vi "OEE_SCREEN_2_update_graph_hourly_data.vi"(11 "SQL_raw_data_out":T1) -> ()   [LabVIEW 2019]
uses:
  FGV/SQL_raw_data/OEE_SQL_raw_data.ctl
  FGV/FGV_SCREEN_2_graph_hourly/FGV_SCREEN_2_graph_hourly.ctl
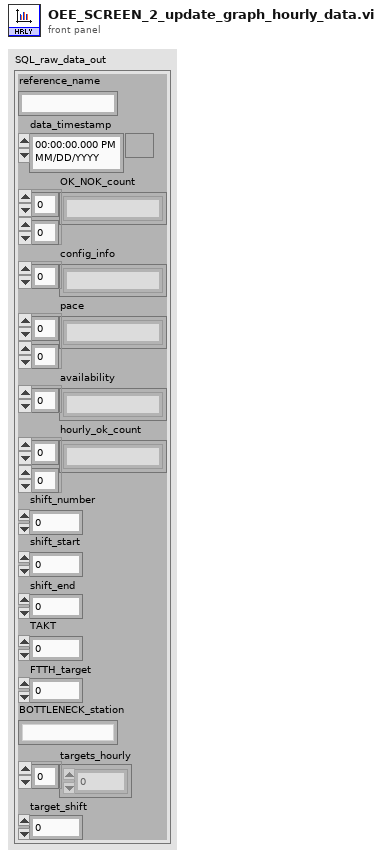
[diagram p1: front panel]
types:
  T1 = typedef "OEE_SQL_raw_data.ctl" = cluster{"reference_name":string, "data_timestamp":timestamp, "OK_NOK_count":string[][], "config_info":string[], "pace":string[][], "availability":string[], "hourly_ok_count":string[][], "shift_number":i8, "shift_start":i8, "shift_end":i8, "TAKT":u16, "FTTH_target":u16, "BOTTLENECK_station":string, "targets_hourly":u16[], "target_shift":u16}
  T2 = typedef "FGV_SCREEN_2_graph_hourly.ctl" = enum16{"initialize", "set_hour_start", "set_hour_end", "set_target", "set_actual", "toggle_visibility", "display"}
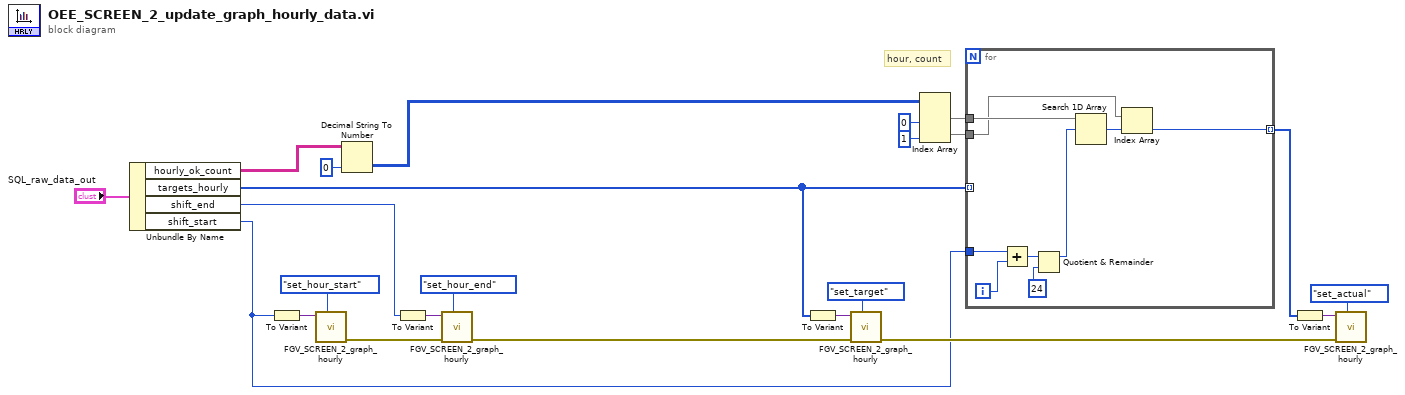
[diagram p0: block diagram]
diagram:
  # "hour, count"
  n1 = Unbundle By Name("SQL_raw_data_out") -> ("hourly_ok_count"=w10:string[][], "targets_hourly"=w1:u16[], "shift_end"=w16:i8, "shift_start"=w4:i8)
  n2 = To Variant(anything=w4) -> (Variant=w18:variant)
  n3 = call "FGV_SCREEN_2_graph_hourly.vi"("options"=FGV_SCREEN_2_graph_hourly."set_hour_start", "input"=w18) -> ("error_out"=w17:errorcluster)  [unwired: 9 in]
  n4 = Decimal String To Number(string=w10, default (0L)=u16 0 ("default (0 I32)")) -> (number=w8:u16[][])  [unwired: 1 in, 1 out]
  n5 = To Variant(anything=w16) -> (Variant=w14:variant)
  n6 = call "FGV_SCREEN_2_graph_hourly.vi"("options"=FGV_SCREEN_2_graph_hourly."set_hour_end", "error_in"=w17, "input"=w14) -> ("error_out"=w12:errorcluster)  [unwired: 8 in]
  n7 = To Variant(anything=w1) -> (Variant=w13:variant)
  n8 = call "FGV_SCREEN_2_graph_hourly.vi"("options"=FGV_SCREEN_2_graph_hourly."set_target", "error_in"=w12, "input"=w13) -> ("error_out"=w23:errorcluster)  [unwired: 8 in]
  n9 = Index Array(array=w8, index (col) #1=0 ("disabled index (col)"), index (col) #2=1 ("index (col)")) -> (element #1=w5:u16[], element #2=w3:u16[])  [unwired: 2 in]
  n10 = for {
    tunnel: w1 -> [_] mode=indexing
    tunnel: w5 -> [w30]
    tunnel: w4 -> [w31]
    tunnel: w3 -> [w28]
    tunnel: [w27] -> w2 mode=indexing
    i -> [w32]
    n11 = Add(x=w31, y=w32) -> (x+y=w26:i32)
    n12 = Quotient & Remainder(x=w26, y=24) -> (x-y*floor(x/y)=w24:i32)  [unwired: 1 out]
    n13 = Search 1D Array(1D array=w30, element=w24) -> (index of element=w29:i32)  [unwired: 1 in]
    n14 = Index Array(array=w28, index=w29) -> (element=w27:u16)
  }
  n15 = To Variant(anything=w2) -> (Variant=w11:variant)
  n16 = call "FGV_SCREEN_2_graph_hourly.vi"("options"=FGV_SCREEN_2_graph_hourly."set_actual", "error_in"=w23, "input"=w11) -> ()  [unwired: 8 in, 1 out]
